vi "Gaussian fitting.vi"(8 "error in (no error)":errorcluster, 10 "above threshold array":bool[](array[boolean]), 11 "Autofocus in":refnum<class "Autofocus.lvclass">) -> (0 "error out":errorcluster, 1 "quality of fit":dbl, 2 "center":dbl, 3 "Autofocus out":refnum<class "Autofocus.lvclass">)   [LabVIEW 2012, in "Autofocus.lvclass"]
uses:
  Autofocus.lvclass
  <vilib>/Analysis/6fits.llb/Curve Fitting Criteria.ctl
  Autofocus.lvclass/Autofocus.ctl
  <userlib>/_OpenG.lib/array/array.llb/Conditional Auto-Indexing Tunnel (DBL)__ogtk.vi
  <vilib>/Analysis/NI_AALPro.lvlib
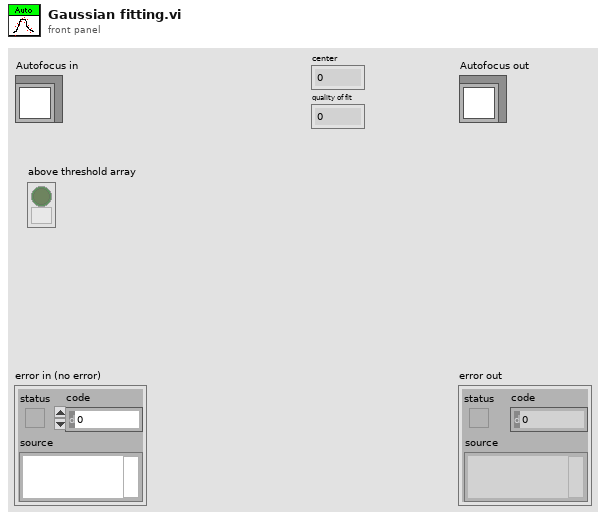
[diagram p1: front panel]
types:
  T1 = cluster{"amp min":dbl, "amp max":dbl, "center min":dbl, "center max":dbl, "deviation min":dbl, "deviation max":dbl, "offset min":dbl, "offset max":dbl}
  T2 = typedef "NI_AALPro.lvlib/Curve Fitting Criteria.ctl" = u16
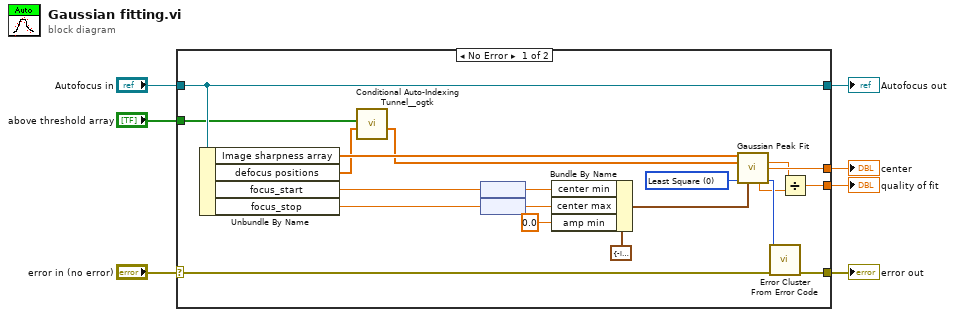
[diagram p0: block diagram]
diagram:
  n1 = case shown="No Error" "error in (no error)" {
    selector: "error in (no error)" -> [w15 w29]
    tunnel: [w14 w29] -> w6
    tunnel: [w27 w28] -> w4
    tunnel: "Autofocus in" -> [w27 w28]
    tunnel: [w17 _] -> w3
    tunnel: [w11 _] -> w2
    tunnel: "above threshold array" -> [w10 _]
    frame No Error {
      w18 = T2 0 items=["Least Square", "Least Absolute Residual", "Bisquare"] ("method")
      n2 = Unbundle By Name(w27) -> ("Image sharpness array"=w26:dbl[], "defocus positions"=w9:dbl[], "focus_start"=w23:dbl[unit], "focus_stop"=w22:dbl[unit])
      n3 = call-poly <userlib>:"Conditional Auto-Indexing Tunnel__ogtk.vi"("Array in"=w9, "Elements to keep"=w10) -> ("Filtered Array out"=w8:dbl[])  [unwired: 5 in]
      n4 = node(w23) -> (w21:dbl)
      n5 = node(w22) -> (w20:dbl)
      n6 = Bundle By Name(cluster=T1 {"amp min"=-inf, "amp max"=inf, "center min"=-inf, "center max"=inf, "deviation min"=-inf, "deviation max"=inf, "offset min"=0.0, "offset max"=0.0} ("parameter bounds"), "center min"=w21, "center max"=w20, "amp min"=0.0) -> (w24:T1)
      n7 = call <vilib>:"Gaussian Peak Fit.vi"("Y"=w26, "X"=w8, "method"=w18, "parameter bounds"=w24) -> ("amplitude"=w13:dbl, "center"=w17:dbl, "residue"=w12:dbl, "error"=w16:i32)  [unwired: 5 in, 3 out]
      n8 = call <vilib>:"Error Cluster From Error Code.vi"("error in (no error)"=w15, "error code (0)"=w16) -> ("error out"=w14:errorcluster)  [unwired: 7 in]
      n9 = Divide(x=w13, y=w12) -> (x/y=w11:dbl)
    }
    frame Error {
    }
  }
  "error out" <- w6
  "Autofocus out" <- w4
  "center" <- w3
  "quality of fit" <- w2
